vi "ArmTeleop.vi"(11 "Setpoint":dbl) -> ()   [LabVIEW 2017]
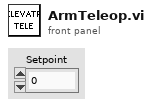
[diagram p1: front panel]
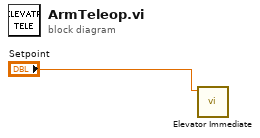
[diagram p0: block diagram]
diagram:
  n1 = call "Elevator Immediate.vi"("Setpoint"="Setpoint") -> ()  [unwired: 10 in, 1 out]
